vi "Callback Change Direction.vi"(6 "Variant":variant, 8 "error in":errorcluster, 9 "Old Values":string[][](array[string]), 10 "object ref in":T2, 11 "Table Change":T3) -> (0 "error out":errorcluster)   [LabVIEW 2013, in "Shared Memory editor node.lvclass"]
doc: "This VI gets called automatically when changes are made to the 'Channel Direction' column of the table and must handle changes appropriately. Register this callback using the appropriate 'Define Column' VI from the Table API."
uses:
  Shared Memory editor node.lvclass
  <vilib>/NI/DCAF/Tag Editor Core/Table API/Table Manager/Cell Change.ctl
  <vilib>/NI/DCAF/Tag Editor Core/Table API/Table Manager/object ref.ctl
  <vilib>/NI/DCAF/Tag Editor Core/Configuration Editor/Classes/Engine Parent/Engine Parent Editor Node.lvclass
  <vilib>/NI/DCAF/Tag Editor Core/Configuration Editor/Classes/Module editor node/module editor node.lvclass
  Permissions Enum.ctl
  module/configuration/Shared Memory configuration.lvclass
  module/configuration/Shared Memory configuration.lvclass/Shared Memory configuration.ctl
  <vilib>/NI/Tag Bus Module Framework/channel/TBM channel.lvclass/TBM channel.ctl
  <vilib>/NI/Configuration Framework/serializable configuration/NISE_CEF_serializable configuration.lvclass/NISE_CEF_serializable configuration.ctl
  <vilib>/Utility/LVClass/Get LV Class Name.vi
  <vilib>/NI/Configuration Framework/error generator/NISE_error generator.vi
  <vilib>/NI/DCAF/Tag Editor Core/Table API/Table Manager.lvlib
  <vilib>/NI/Tag Bus Module Framework/channel/TBM channel.lvclass
  <vilib>/NI/Configuration Framework/serializable configuration/NISE_CEF_serializable configuration.lvclass
  <vilib>/NI/Module Execution Interface/Engine Configuration/engine configuration.lvclass
  <vilib>/NI/DCAF/Tag Editor Core/Table API/Table Manager/Table Manager.lvclass
panel:
  in  "Permissions":T1=enum."Read from Memory"
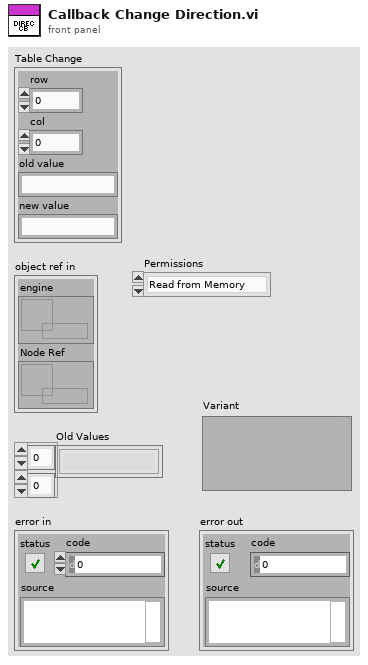
[diagram p1: front panel]
types:
  T1 = typedef "Shared Memory editor node.lvclass/Permissions Enum.ctl" = enum16{"Write to Memory", "Read from Memory"}
  T2 = typedef "Table Manager.lvlib/Table Manager.lvclass/object ref.ctl" = cluster{"engine":refnum<data-value>, "Node Ref":refnum<data-value>}
  T3 = typedef "Table Manager.lvlib/Cell Change.ctl" = cluster{"row":i32, "col":i32, "old value":string, "new value":string}
  T4 = typedef "Shared Memory configuration.lvclass/Line.ctl" = cluster{"channel":refnum<class "TBM channel.lvclass">}
  T5 = typedef "TBM channel.lvclass/channel classification.ctl" = enum16{"input data", "output data", "processing parameter", "processing result"}
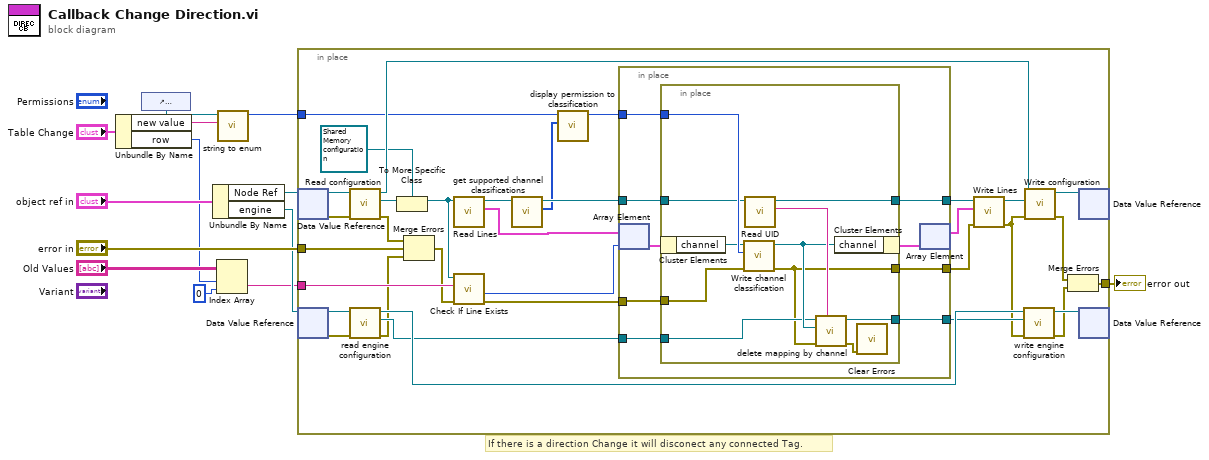
[diagram p0: block diagram]
diagram:
  # "If there is a direction Change it will disconect any connected Tag."
  n1 = Unbundle By Name("Table Change") -> ("new value"=w2:string, "row"=w3:i32)
  n2 = control-ref of="Permissions"() -> (w7:refnum<vi>)
  n3 = Unbundle By Name("object ref in") -> ("Node Ref"=w10:refnum<data-value>, "engine"=w9:refnum<data-value>)
  n4 = Index Array(array="Old Values", index (row)=w3, index (col)=0 ("disabled index (col)")) -> (element=w4:string)
  n5 = call <vilib>:"string to enum.vi"("String"=w2, "Enum"=w7) -> ("Value"=w1:i32)  [unwired: 8 in, 1 out]
  n6 = in-place {
    in-place-border: [w40] -> w13
    in-place-border: "error in" -> [w20]
    in-place-border: w1 -> [w16]
    in-place-border: w4 -> [w28]
    n7 = in-place-dvr #1(w10) -> (w37:refnum<class "module editor node.lvclass">, w39:errorcluster)
    n8 = in-place-dvr #2(w9) -> (w46:refnum<class "Engine Parent Editor Node.lvclass">, w47:errorcluster)
    n9 = call-dynamic "Read configuration.vi"("error in"=w39, "NISE_CEF_serializable node in"=w37) -> ("error out"=w38:errorcluster, "configuration"=w35:refnum<class "NISE_CEF_serializable configuration.lvclass">, "NISE_CEF_serializable node out"=w36:refnum<class "module editor node.lvclass">)  [unwired: 7 in]
    n10 = call <vilib>:"read engine configuration.vi"("error in"=w47, "Engine Parent Editor Node in"=w46) -> ("error out"=w19:errorcluster, "engine configuration"=w26:refnum<class "engine configuration.lvclass">, "Engine Parent Editor Node out"=w43:refnum<class "Engine Parent Editor Node.lvclass">)  [unwired: 7 in]
    n11 = To More Specific Class(target class=refnum<class "Shared Memory configuration.lvclass"> refnum ("tag bus configurable plugin module configuration"), reference=w35) -> (specific class reference=w32:refnum<class "Shared Memory configuration.lvclass">)  [unwired: 1 in, 1 out]
    n12 = Merge Errors(w38, w20, w19) -> (w24:errorcluster)
    n13 = call "Read Lines.vi"("Shared Memory configuration in"=w32) -> ("Lines"=w31:T4[], "Shared Memory configuration out"=w18:refnum<class "Shared Memory configuration.lvclass">)  [unwired: 8 in, 1 out]
    n14 = call-dynamic "Check If Line Exists.vi"("error in"=w24, "Name to Locate"=w28, "Shared Memory configuration in"=w32) -> ("error out"=w23:errorcluster, "Index"=w29:i32)  [unwired: 4 in, 3 out]
    n15 = call-dynamic "get supported channel classifications.vi"("module configuration in"=w18) -> ("supported classes"=w14:T5[], "module configuration out"=w17:refnum<class "Shared Memory configuration.lvclass">)  [unwired: 8 in, 1 out]
    n16 = call "display permission to classification.vi"("supported classes"=w14, "display permissions"=w16) -> ("channel classification"=w15:T5)  [unwired: 9 in]
    n17 = in-place {
      in-place-border: w15 -> [w54]
      in-place-border: w17 -> [w53]
      in-place-border: [w52] -> w27
      in-place-border: w26 -> [w51]
      in-place-border: [w50] -> w25
      in-place-border: w23 -> [w49]
      in-place-border: [w48] -> w22
      n18 = in-place-array #3(w31, w29) -> (w56:T4)
      n19 = in-place {
        in-place-border: w54 -> [w67]
        in-place-border: w53 -> [w66]
        in-place-border: [w65] -> w52
        in-place-border: w51 -> [w59]
        in-place-border: [w63] -> w50
        in-place-border: w49 -> [w60]
        in-place-border: [w57] -> w48
        n20 = in-place-cluster #4(w56) -> ("channel"=w64:refnum<class "TBM channel.lvclass">)
        n21 = call <vilib>:"Write channel classification.vi"("error in"=w60, "channel classification"=w67, "channel in"=w64) -> ("error out"=w57:errorcluster, "channel out"=w61:refnum<class "TBM channel.lvclass">)  [unwired: 7 in]
        n22 = call <vilib>:"Read UID.vi"("configuration in"=w66) -> ("instance id"=w62:string, "configuration out"=w65:refnum<class "Shared Memory configuration.lvclass">)  [unwired: 8 in, 1 out]
        n23 = call <vilib>:"delete mapping by channel.vi"("owner ID"=w62, "error in"=w57, "channel"=w61, "engine configuration in"=w59) -> ("error out"=w58:errorcluster, "engine configuration out"=w63:refnum<class "engine configuration.lvclass">)  [unwired: 6 in]
        n24 = in-place-cluster #4("channel"=w61) -> (w55:T4)
        n25 = call <vilib>:"Clear Errors.vi"("error in (no error)"=w58) -> ()  [unwired: 6 in, 1 out]
      }
      n26 = in-place-array #3(w55) -> (w30:T4[])  [unwired: 1 out]
    }
    n27 = call "Write Lines.vi"("error in (no error)"=w22, "Lines"=w30, "Shared Memory configuration in"=w27) -> ("error out"=w21:errorcluster, "Shared Memory configuration out"=w33:refnum<class "Shared Memory configuration.lvclass">)  [unwired: 7 in]
    n28 = call <vilib>:"write engine configuration.vi"("error in"=w21, "engine configuration"=w25, "Engine Parent Editor Node in"=w43) -> ("error out"=w42:errorcluster, "Engine Parent Editor Node out"=w45:refnum<class "Engine Parent Editor Node.lvclass">)  [unwired: 7 in]
    n29 = call-dynamic "Write configuration.vi"("error in"=w21, "configuration"=w33, "NISE_CEF_serializable node in"=w36) -> ("error out"=w41:errorcluster, "NISE_CEF_serializable node out"=w44:refnum<class "module editor node.lvclass">)  [unwired: 7 in]
    n30 = Merge Errors(w41, w42) -> (w40:errorcluster)
    n31 = in-place-dvr #1(w44) -> ()  [unwired: 2 out]
    n32 = in-place-dvr #2(w45) -> ()  [unwired: 2 out]
  }
  "error out" <- w13
